vi "Read out POLARITY.vi"(5 "All Channels (T)":bool=TRUE, 7 "Channel":u8, 8 "error in (no error)":errorcluster, 11 "BoardHandle":T1) -> (0 "error out":errorcluster, 2 "Polarity values":string[](array[string]), 3 "BoardHandle out":T1)   [LabVIEW 2009, in "CAEN PSM.lvlib"]
doc: "This function returns channels polarity"
uses:
  <instrlib>/CAEN PSM/CAEN PSM.lvlib
  <instrlib>/CAEN PSM/Private/BoardHandle.ctl
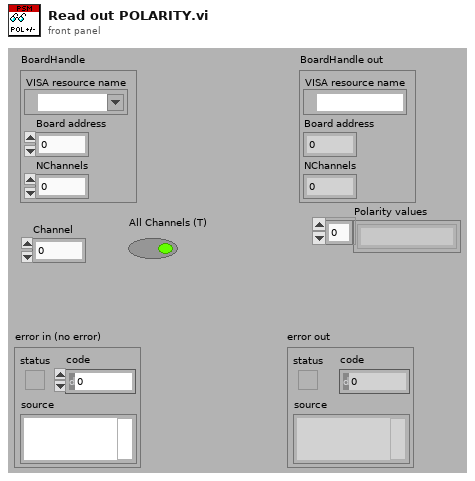
[diagram p1: front panel]
types:
  T1 = typedef "CAEN PSM.lvlib/BoardHandle.ctl" = cluster{"VISA resource name":refnum<visa-resource-name>, "Board address":u8, "NChannels":u8}
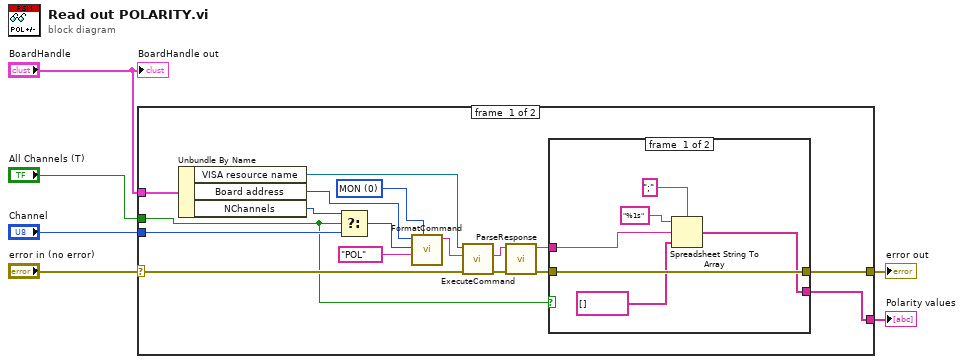
[diagram p0: block diagram]
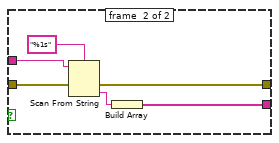
[diagram p2: hidden frame]
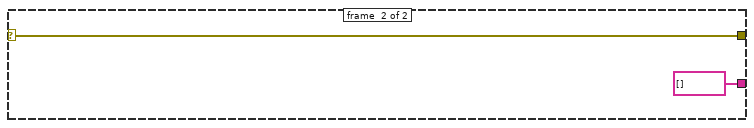
[diagram p3: hidden frame]
diagram:
  n1 = case shown="No Error" "error in (no error)" {
    selector: "error in (no error)" -> [w14 w37]
    tunnel: "All Channels (T)" -> [w7 _]
    tunnel: "Channel" -> [w21 _]
    tunnel: [w9 w37] -> w3
    tunnel: "BoardHandle" -> [w15 _]
    tunnel: [w8 string[] []] -> w1
    frame #0 {
      w22 = u8 0 items=["MON", "SET"] ("CMD")
      n2 = Unbundle By Name(w15) -> ("VISA resource name"=w19:refnum<visa-resource-name>, "Board address"=w23:u8, "NChannels"=w12:u8)
      n3 = Select(t=w12, s=w7, f=w21) -> (s? t:f=w20:u8)
      n4 = call <instrlib>:"FormatCommand.vi"("CMD (MON)"=w22, "PAR"="POL", "CH"=w20, "BD (0)"=w23) -> ("cmd"=w18:string)  [unwired: 7 in]
      n5 = call <instrlib>:"ExecuteCommand.vi"("error in (no error)"=w14, "Command"=w18, "VISA resource name"=w19) -> ("error out"=w17:errorcluster, "Response"=w16:string)  [unwired: 6 in, 1 out]
      n6 = call <instrlib>:"ParseResponse.vi"("error in (no error)"=w17, "Response"=w16) -> ("error out"=w10:errorcluster, "val"=w11:string)  [unwired: 6 in, 2 out]
      n7 = case shown="True" w7 {
        tunnel: w11 -> [w26 w35]
        tunnel: w10 -> [w29 w33]
        tunnel: [w29 w32] -> w9
        tunnel: [w24 w30] -> w8
        frame #0 {
          n8 = Spreadsheet String To Array(delimiter (Tab)=";", format string="%1s", spreadsheet string=w26, array type (2D Dbl)=string[] []) -> (array=w24:string[])
        }
        frame #1 {
          n9 = Scan From String(format string="%1s", input string=w35, error in=w33) -> (error out=w32:errorcluster, output 1=w31:string)  [unwired: 2 in, 2 out]
          n10 = Build Array(w31) -> (w30:string[])
        }
      }
    }
    frame #1 {
    }
  }
  "error out" <- w3
  "Polarity values" <- w1
  "BoardHandle out" <- "BoardHandle"
